vi "GetAlarms.vi"(0 "Engine_1DO_2DI in":refnum<class "Engine_1DO_2DI.lvclass">, 11 "error in (no error)":errorcluster) -> (4 "Engine_1DO_2DI out":refnum<class "Engine_1DO_2DI.lvclass">, 6 "Alarm":bool, 8 "Warning":bool, 15 "error out":errorcluster)   [LabVIEW 2019, in "Engine_1DO_2DI.lvclass"]
uses:
  Engine_1DO_2DI.lvclass
  Engine_1DO_2DI.lvclass/Engine_1DO_2DI.ctl
  DA_class/DA.lvclass
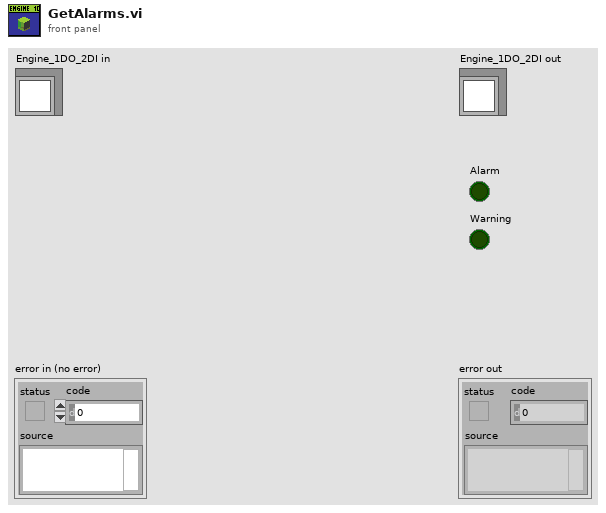
[diagram p1: front panel]
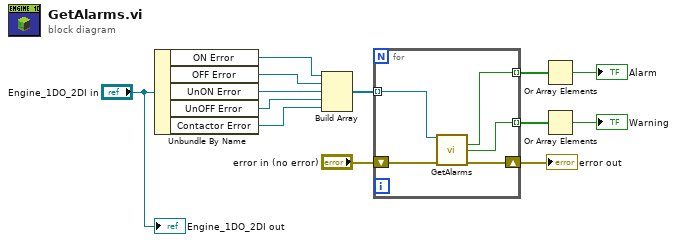
[diagram p0: block diagram]
diagram:
  n1 = Unbundle By Name("Engine_1DO_2DI in") -> ("ON Error"=w13:refnum<class "DA.lvclass">, "OFF Error"=w12:refnum<class "DA.lvclass">, "UnON Error"=w11:refnum<class "DA.lvclass">, "UnOFF Error"=w10:refnum<class "DA.lvclass">, "Contactor Error"=w9:refnum<class "DA.lvclass">)
  n2 = Build Array(w13, w12, w11, w10, w9) -> (w8:refnum<class "DA.lvclass">[])
  n3 = for {
    tunnel: w8 -> [w18] mode=indexing
    tunnel: [w17] -> w7 mode=indexing
    tunnel: [w16] -> w6 mode=indexing
    shift-right: [w15] -> w3
    shift-left: "error in (no error)" -> [w14]
    n4 = call-dynamic "GetAlarms.vi"("DA in"=w18, "error in (no error)"=w14) -> ("Alarm"=w17:bool, "Warning"=w16:bool, "error out"=w15:errorcluster)  [unwired: 10 in, 1 out]
  }
  "error out" <- w3
  n5 = Or Array Elements(Boolean array=w7) -> (logical OR=→"Alarm":bool)
  n6 = Or Array Elements(Boolean array=w6) -> (logical OR=→"Warning":bool)
  "Engine_1DO_2DI out" <- "Engine_1DO_2DI in"
